vi "Measure.vi"() -> ()   [LabVIEW 2012]
uses:
  Controls/TestData.ctl
  Controls/TestArea.ctl
  Classes/Instruments.lvclass
panel:
  in  "Cluster 3":T3 {"TestData"."50mA Data"."Current,mA" format="%_6g"; "TestData"."50mA Data"."WL" format="%_6g"; "TestData"."50mA Data"."Voltage" format="%_6g"; "TestData"."50mA Data"."Power" format="%_6g"; "TestData"."20mA Data"."Reverse" format="%#_3g"; "TestData"."20mA Data"."Current,mA" format="%_6g"; "TestData"."20mA Data"."Knee Current" format="%#_3g"; "TestData"."20mA Data"."WL" format="%_6g"; "TestData"."20mA Data"."Voltage" format="%_6g"; "TestData"."20mA Data"."Power" format="%_5g"}
  out "Data Out":T2 {"50mA Data"."Current,mA" format="%_6g"; "50mA Data"."WL" format="%_6g"; "50mA Data"."Voltage" format="%_6g"; "50mA Data"."Power" format="%_6g"; "20mA Data"."Reverse" format="%#_3g"; "20mA Data"."Current,mA" format="%_6g"; "20mA Data"."Knee Current" format="%#_3g"; "20mA Data"."WL" format="%_6g"; "20mA Data"."Voltage" format="%_6g"; "20mA Data"."Power" format="%_5g"}
  # "Current Result"
  # "Measure Control"
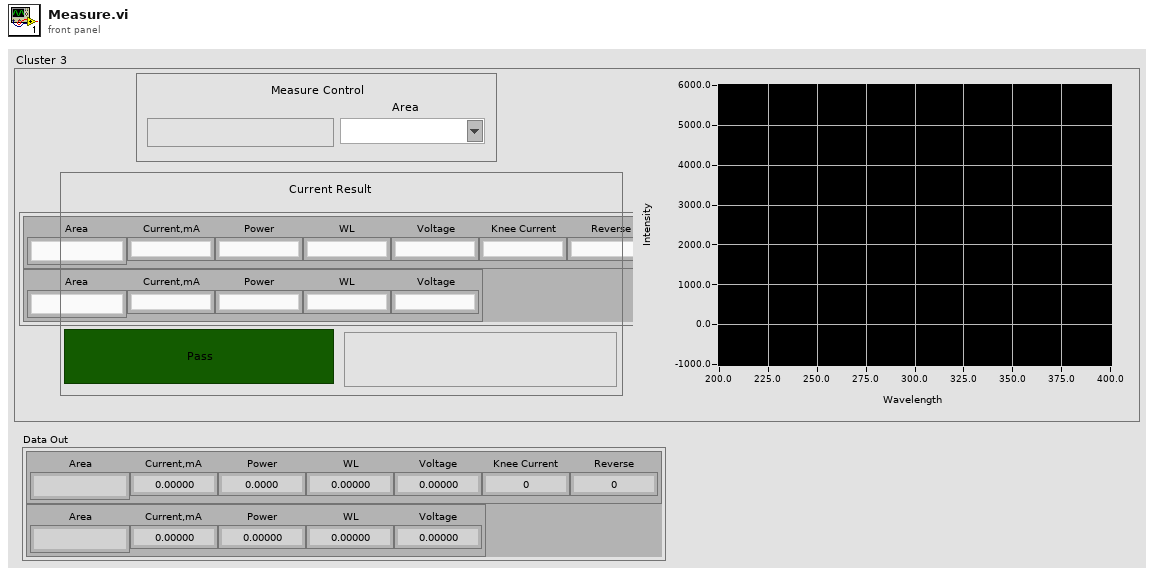
[diagram p1: front panel]
types:
  T1 = typedef "TestArea.ctl" = string
  T2 = typedef "TestData.ctl" = cluster{"20mA Data":cluster{"Area":string, "Current,mA":dbl, "Power":dbl, "WL":dbl, "Voltage":dbl, "Knee Current":dbl, "Reverse":dbl}, "50mA Data":cluster{"Area":string, "Current,mA":dbl, "Power":dbl, "WL":dbl, "Voltage":dbl}}
  T3 = cluster{"Pass":bool, "Fail":bool, "Measure":bool, "Area":T1, "TestData":T2, "XY Graph":cluster{"Y":dbl[], "Y":dbl[]}[]}
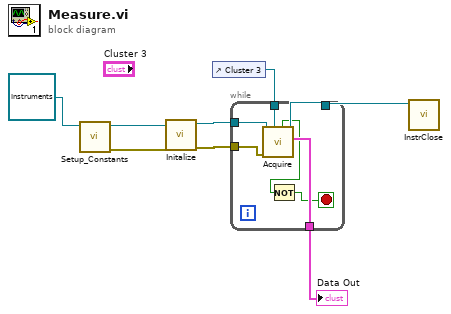
[diagram p0: block diagram]
diagram:
  n1 = call-dynamic "Setup_Constants.vi"("Instruments in"=refnum<class "Instruments.lvclass"> refnum ("Instruments.lvclass")) -> ("error out"=w3:errorcluster, "Instruments out"=w7:refnum<class "Instruments.lvclass">)  [unwired: 9 in]
  n2 = call-dynamic "Initalize.vi"("error in (no error)"=w3, "Instruments in"=w7) -> ("error out"=w4:errorcluster, "Instruments out"=w6:refnum<class "Instruments.lvclass">)  [unwired: 8 in]
  n3 = control-ref of="Cluster 3"() -> (w1:refnum<vi>)
  n4 = while {
    tunnel: w6 -> [w15]
    tunnel: [w14] -> w5
    tunnel: w4 -> [w13]
    tunnel: [w12] -> w2
    tunnel: w1 -> [w11]
    stop <- w9 stop-if-true
    n5 = call-dynamic "Acquire.vi"("MeasureControl"=w11, "error in (no error)"=w13, "Instruments in"=w15) -> ("Data Out"=w14:T2, "Instruments out"=w12:refnum<class "Instruments.lvclass">, "Overrange"=w10:bool)  [unwired: 3 in, 3 out]
    n6 = Not(x=w10) -> (.not. x?=w9:bool)
  }
  "Data Out" <- w5
  n7 = call-dynamic "InstrClose.vi"("Instruments in"=w2) -> ()  [unwired: 9 in, 2 out]
